vi "Open.vi"(8 "error in (no error)":errorcluster, 11 "Logfile":path) -> (0 "error out":errorcluster, 3 "Logfile Ref Out":refnum<file>)   [LabVIEW 2016, in "Log4Lv.lvlib"]
doc: "Use this template to build a VI to use as a subVI."
uses:
  Log4Lv.lvlib
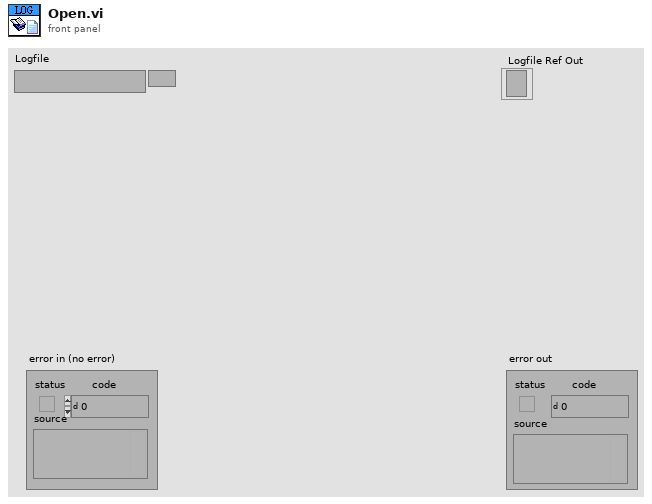
[diagram p1: front panel]
types:
  T1 = enum16{"open", "replace", "create", "open or create", "replace or create", "replace or create with confirmation"}
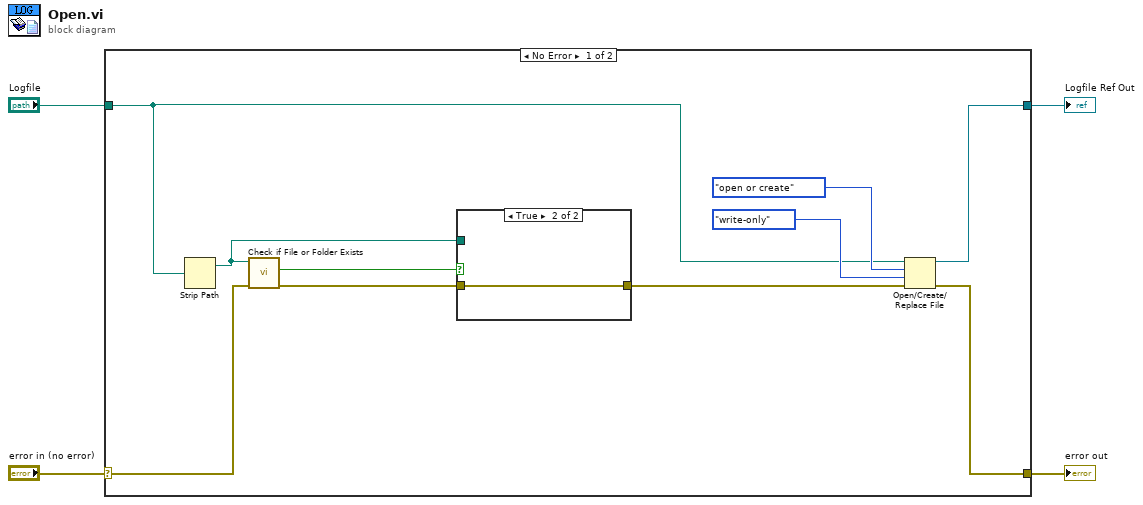
[diagram p0: block diagram]
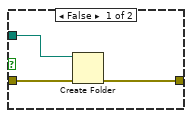
[diagram p2: hidden frame]
diagram:
  n1 = case shown="No Error" "error in (no error)" {
    selector: "error in (no error)" -> [w8 w19]
    tunnel: [w13 w19] -> w3
    tunnel: "Logfile" -> [w5 _]
    tunnel: [w14 _] -> w1
    frame No Error {
      n2 = Strip Path(path=w5) -> (stripped path=w9:path)  [unwired: 1 out]
      n3 = call <vilib>:"Check if File or Folder Exists.vi"("error in (no error)"=w8, "path"=w9) -> ("error out"=w7:errorcluster, "file or folder exists?"=w10:bool)  [unwired: 7 in, 1 out]
      n4 = case shown="True" w10 {
        tunnel: w9 -> [w17 _]
        tunnel: w7 -> [w16 w18]
        tunnel: [w15 w18] -> w6
        frame False {
          n5 = Create Folder(path (use dialog)=w17, error in=w16) -> (error out=w15:errorcluster)  [unwired: 1 in, 2 out]
        }
        frame True {
        }
      }
      n6 = Open/Create/Replace File(file path (use dialog)=w5, error in=w6, operation (0:open)=T1."open or create", access (0:read/write)=enum16{"read/write", "read-only", "write-only"}."write-only") -> (refnum out=w14:refnum<file>, error out=w13:errorcluster)  [unwired: 2 in, 1 out]
    }
    frame Error {
    }
  }
  "error out" <- w3
  "Logfile Ref Out" <- w1
